vi "open.vi"(8 "error in (no error)":errorcluster caption="错误输入（无错误）", 10 "database":string, 11 "access 输入":refnum<class "access.lvclass">) -> (0 "error out":errorcluster caption="错误输出", 3 "access 输出":refnum<class "access.lvclass">)   [LabVIEW 2016, in "潮位站数据传输.lvlib" / "access.lvclass"]
uses:
  access.lvclass
  <vilib>/Utility/sysdir.llb/System Directory Type.ctl
  database_class/database.lvclass/database.ctl
  <vilib>/addons/database/Connection.llb/DB Tools Open Connec (String).vi
  <vilib>/addons/database/NI_Database_API.lvlib
  database_class/database.lvclass
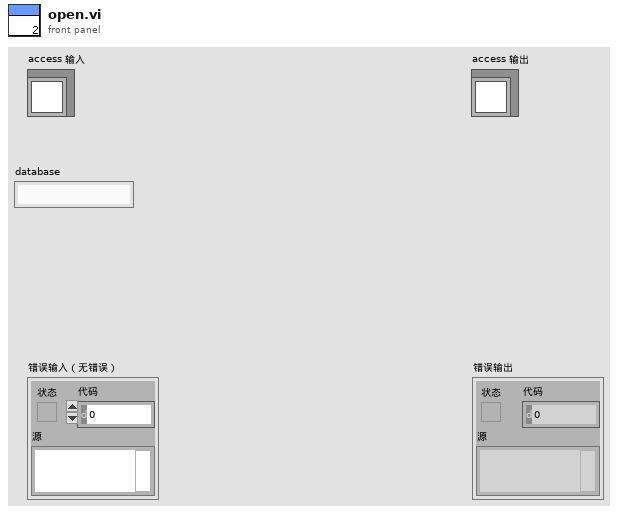
[diagram p1: front panel]
types:
  T1 = typedef "System Directory Type.ctl" = i32
  T2 = typedef "NI_Database_API.lvlib/Conn ObjectReference.ctl" = refnum<k1>
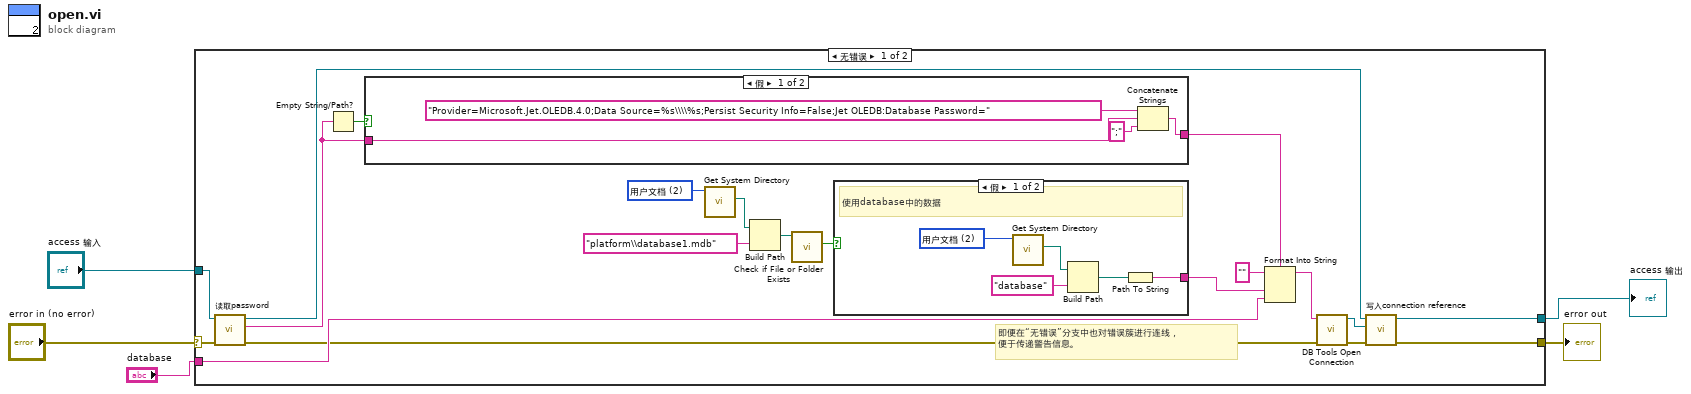
[diagram p0: block diagram]
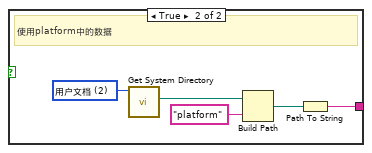
[diagram p2: hidden frame]
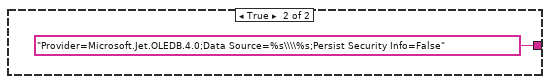
[diagram p3: hidden frame]
diagram:
  n1 = case shown="无错误" "error in (no error)" {
    selector: "error in (no error)" -> [w12 w41]
    tunnel: "access 输入" -> [w14 w42]
    tunnel: [w8 w42] -> w5
    tunnel: "database" -> [w15 _]
    tunnel: [w6 w41] -> w3
    frame No Error {
      w22 = T1 2 items=["用户目录"=0, "用户桌面"=1, "用户文档"=2, "用户应用程序数据"=3, "用户设置"=4, "用户临时目录"=5, "公共文档"=6, "公共应用程序数据"=7, "公共设置"=8, "公共缓存"=13, "系统核心库"=9, "系统安装库"=10, "应用程序文件"=11, "启动盘根目录"=12] ("system directory type")
      # "即便在“无错误”分支中也对错误簇进行连线，\n便于传递警告信息。"
      n2 = call "读取password.vi"("error in (no error)"=w12, "database输入"=w14) -> ("error out"=w11:errorcluster, "password"=w13:string, "database输出"=w10:refnum<class "access.lvclass">)  [unwired: 7 in]
      n3 = Empty String/Path?(string/path=w13) -> (empty?=w25:bool)
      n4 = case shown="假" w25 {
        tunnel: [w36 "Provider=Microsoft.Jet.OLEDB.4.0;Data Source=%s\\\\%s;Persist Security Info=False" ("格式字符串")] -> w17
        tunnel: w13 -> [w39 _]
        frame False {
          n5 = Concatenate Strings("Provider=Microsoft.Jet.OLEDB.4.0;Data Source=%s\\\\%s;Persist Security Info=False;Jet OLEDB:Database Password=" ("格式字符串"), w39, ";" ("字符串")) -> (w36:string)
        }
        frame True {
        }
      }
      n6 = call <vilib>:"Get System Directory.vi"("system directory type"=w22) -> ("system directory"=w23:path)  [unwired: 10 in]
      n7 = Build Path(base path=w23, name or relative path="platform\\database1.mdb" ("condition")) -> (appended path=w21:path)
      n8 = call <vilib>:"Check if File or Folder Exists.vi"("path"=w21) -> ("file or folder exists?"=w19:bool)  [unwired: 8 in, 2 out]
      n9 = case shown="假" w19 {
        tunnel: [w26 w31] -> w18
        frame False {
          w29 = T1 2 items=["用户目录"=0, "用户桌面"=1, "用户文档"=2, "用户应用程序数据"=3, "用户设置"=4, "用户临时目录"=5, "公共文档"=6, "公共应用程序数据"=7, "公共设置"=8, "公共缓存"=13, "系统核心库"=9, "系统安装库"=10, "应用程序文件"=11, "启动盘根目录"=12] ("system directory type")
          # "使用database中的数据"
          n10 = call <vilib>:"Get System Directory.vi"("system directory type"=w29) -> ("system directory"=w28:path)  [unwired: 10 in]
          n11 = Build Path(base path=w28, name or relative path="database" ("condition")) -> (appended path=w30:path)
          n12 = Path To String(path=w30) -> (string=w26:string)
        }
        frame True {
          w35 = T1 2 items=["用户目录"=0, "用户桌面"=1, "用户文档"=2, "用户应用程序数据"=3, "用户设置"=4, "用户临时目录"=5, "公共文档"=6, "公共应用程序数据"=7, "公共设置"=8, "公共缓存"=13, "系统核心库"=9, "系统安装库"=10, "应用程序文件"=11, "启动盘根目录"=12] ("system directory type")
          # "使用platform中的数据"
          n13 = call <vilib>:"Get System Directory.vi"("system directory type"=w35) -> ("system directory"=w34:path)  [unwired: 10 in]
          n14 = Build Path(base path=w34, name or relative path="platform" ("condition")) -> (appended path=w32:path)
          n15 = Path To String(path=w32) -> (string=w31:string)
        }
      }
      n16 = Format Into String(format string=w17, initial string="" ("初始字符串"), w18, w15) -> (resulting string=w16:string)  [unwired: 1 in, 1 out]
      n17 = call-poly <vilib>:"DB Tools Open Connection.vi"("error in (no error)"=w11, "connection information"=w16) -> ("error out"=w7:errorcluster, "connection reference"=w9:T2)  [unwired: 6 in]
      n18 = call-dynamic "写入connection reference.vi"("error in (no error)"=w7, "reference"=w9, "database输入"=w10) -> ("error out"=w6:errorcluster, "database输出"=w8:refnum<class "access.lvclass">)  [unwired: 7 in]
    }
    frame Error {
    }
  }
  "error out" <- w3
  "access 输出" <- w5
